vi "GetDataFromMain.vi"() -> (2 "SN":string, 3 "Profile":string)   [LabVIEW 2020]
uses:
  <vilib>/Utility/config.llb/Read Key (String).vi
  <vilib>/Utility/config.llb/NI_LVConfig.lvlib
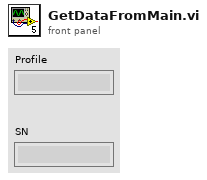
[diagram p1: front panel]
types:
  T1 = typedef "NI_LVConfig.lvlib/Config Data RefNum.ctl" = refnum<k1>
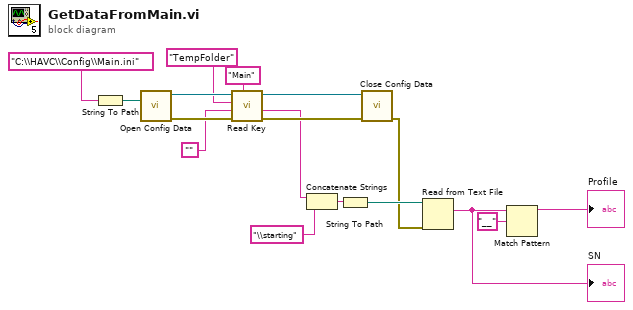
[diagram p0: block diagram]
diagram:
  n1 = String To Path(string="C:\\HAVC\\Config\\Main.ini") -> (path=w17:path)
  n2 = call <vilib>:"Open Config Data.vi"("configuration file path"=w17) -> ("error out"=w14:errorcluster, "refnum"=w13:T1)  [unwired: 8 in, 1 out]
  n3 = call-poly <vilib>:"Read Key.vi"("section"="Main", "error in (no error)"=w14, "default value"="", "key"="TempFolder", "refnum"=w13) -> ("error out"=w15:errorcluster, "value"=w7:string, "refnum out"=w12:T1)  [unwired: 3 in, 1 out]
  n4 = Concatenate Strings(w7, "\\starting") -> (w6:string)
  n5 = String To Path(string=w6) -> (path=w5:path)
  n6 = call <vilib>:"Close Config Data.vi"("error in (no error)"=w15, "refnum"=w12) -> ("error out"=w4:errorcluster)  [unwired: 8 in, 1 out]
  n7 = Read from Text File(file (use dialog)=w5, error in=w4) -> (text=w3:string)  [unwired: 2 in, 3 out]
  "SN" <- w3
  n8 = Match Pattern(string=w3, regular expression="__") -> (before substring=→"Profile":string)  [unwired: 1 in, 3 out]
